vi "New Startup.vi"   [LabVIEW 2013]
uses:
  user/michelle/QDServer/QDServGlobal.vi
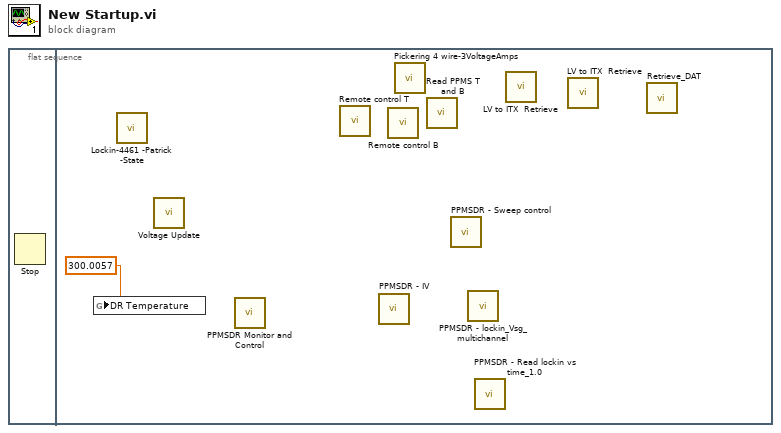
[diagram p0: block diagram]
diagram:
  n1 = flat-sequence {
    frame #0 {
      n2 = Stop() -> ()  [unwired: 1 in]
    }
    frame #1 {
      n3 = global write "QDServGlobal.vi" "DR Temperature"(300.0057 ("DR Temperature")) -> ()
      n4 = call <userlib>:"Lockin-4461 -Patrick -State.vi"() -> ()  [unwired: 12 in]
      n5 = call <userlib>:"Voltage Update.vi"() -> ()  [unwired: 9 in]
      n6 = call "PPMSDR Monitor and Control.vi"() -> ()  [unwired: 12 in]
      n7 = call <vilib>:"Remote control T.vi"() -> ()  [unwired: 6 in]
      n8 = call "PPMSDR - IV.vi"() -> ()  [unwired: 12 in]
      n9 = call <userlib>:"Remote control B.vi"() -> ()  [unwired: 9 in, 1 out]
      n10 = call <userlib>:"Pickering 4 wire-3VoltageAmps.vi"() -> ()  [unwired: 12 in]
      n11 = call <userlib>:"Read PPMS T and B.vi"() -> ()  [unwired: 3 in, 3 out]
      n12 = call "PPMSDR - Sweep control.vi"() -> ()  [unwired: 9 in]
      n13 = call "PPMSDR - lockin_Vsg_multichannel.vi"() -> ()  [unwired: 12 in]
      n14 = call "PPMSDR - Read lockin vs time_1.0.vi"() -> ()  [unwired: 9 in, 3 out]
      n15 = call <userlib>:"LV to ITX  Retrieve.vi"() -> ()  [unwired: 11 in, 5 out]
      n16 = call <userlib>:"LV to ITX  Retrieve.vi"() -> ()  [unwired: 11 in, 5 out]
      n17 = call "Retrieve_DAT.vi"() -> ()  [unwired: 12 in]
    }
  }
